vi "matrici_v51.vi"() -> ()   [LabVIEW 2009]
uses:
  <vilib>/Math Plots/3D Math Plots/3D Surface/3D Surface XCtrl/3D Surface.xctl
  <vilib>/Math Plots/3D Math Plots/3D Surface/3D Surface Datatype/3D Surface Datatype.lvclass
  <vilib>/Math Plots/3D Math Plots/3D Surface/3D Surface Datatype/Public/Plot Helper (Vector).vi
panel:
  in  "eps":dbl(slide)=68.57142857142857 scale=0.0..80.0
  in  "sig":dbl(slide)=0.5737051792828685 scale=0.0..2.0
  out "3D Surface":refnum<class "3D Plot Datatype.lvclass">[](xcontrol)
  out "X":dbl=11.655138339920956
  out "y":dbl=11.655138339920956
  in  "stop":bool
  in  "Domeniul de definitie x,y":dbl(slide)=23.3102766798419 scale=0.5..100.0
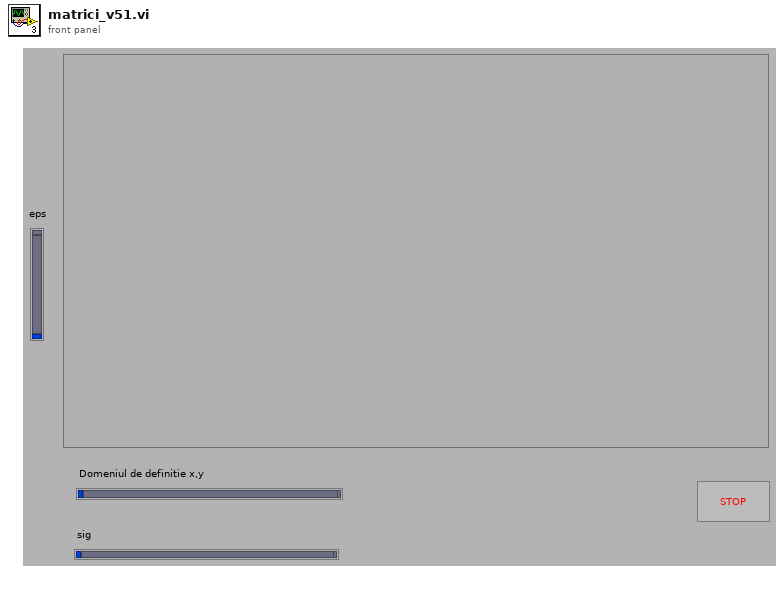
[diagram p1: front panel]
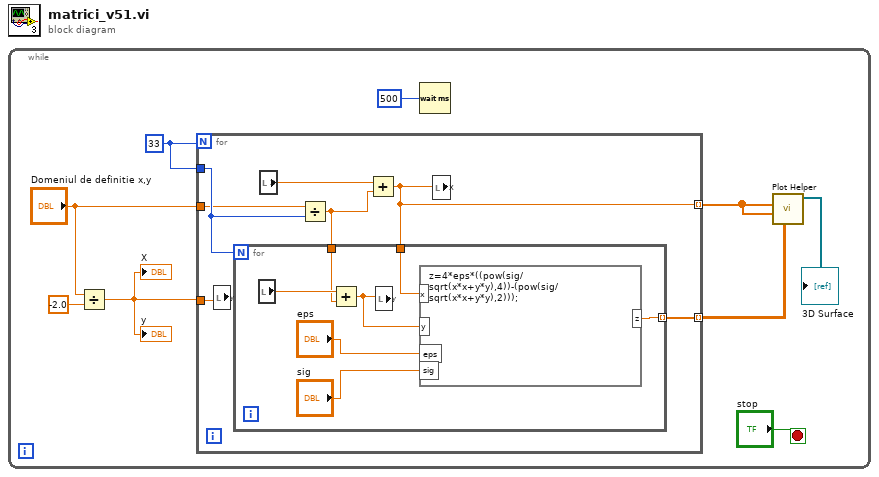
[diagram p0: block diagram]
diagram:
  n1 = while {
    stop <- "stop" stop-if-true
    w5 = 33
    n2 = Divide(x="Domeniul de definitie x,y", y=-2.0) -> (x/y=w2:dbl)
    "X" <- w2
    "y" <- w2
    n3 = for {
      N: w5 -> [_]
      tunnel: [w15] -> w9 mode=indexing
      tunnel: [w14] -> w1 mode=indexing
      tunnel: w5 -> [w13]
      tunnel: w2 -> [w11]
      tunnel: "Domeniul de definitie x,y" -> [w10]
      n4 = local write "y"(w11) -> ()
      n5 = local read "X"() -> (w16:dbl)
      n6 = Divide(x=w10, y=w13) -> (x/y=w12:dbl)
      n7 = Add(x=w16, y=w12) -> (x+y=w15:dbl)
      n8 = for {
        N: w13 -> [_]
        tunnel: w15 -> [w22]
        tunnel: [w20] -> w14 mode=indexing
        tunnel: w12 -> [w19]
        n9 = local read "y"() -> (w23:dbl)
        n10 = Add(x=w23, y=w19) -> (x+y=w21:dbl)
        n11 = local write "y"(w21) -> ()
        n12 = formula code="z=4*eps*((pow(sig/sqrt(x*x+y*y),4))-(pow(sig/sqrt(x*x+y*y),2)));"("x"=w22, "y"=w21, "eps"="eps", "sig"="sig") -> ("z"=w20:dbl)
      }
      n13 = local write "X"(w15) -> ()
    }
    n14 = Wait (ms)(milliseconds to wait=500) -> ()  [unwired: 1 out]
    n15 = call-poly <vilib>:"Plot Helper.vi"("z matrix"=w1, "y vector"=w9, "x vector"=w9) -> ("3D Plot lvclass Array out"=→"3D Surface":refnum<class "3D Plot Datatype.lvclass">[])  [unwired: 3 in, 5 out]
  }
